vi "Seg_2_discharging.vi"(0 "VISA Refnum in":refnum<visa-resource-name>, 1 "Log??":bool, 2 "File_name":string, 5 "Numeric":i32, 7 "Index":i32, 9 "Discharge Stop Voltage":dbl=3.5 format="%#_13g", 11 "error in (no error)":errorcluster) -> (3 "Stop discharging":bool, 4 "VISA Refnum out":refnum<visa-resource-name>, 6 "Curent Tracking 2":dbl caption="Curent Tracking" format="%.8f", 10 "Voltage Tracking 2":dbl caption="Voltage Tracking" format="%.8f", 15 "error out":errorcluster)   [LabVIEW 2015]
uses:
  <vilib>/Utility/file.llb/Write Delimited Spreadsheet (string).vi
  <instrlib>/Agilent N6700 Series/Agilent N6700 Series.lvlib
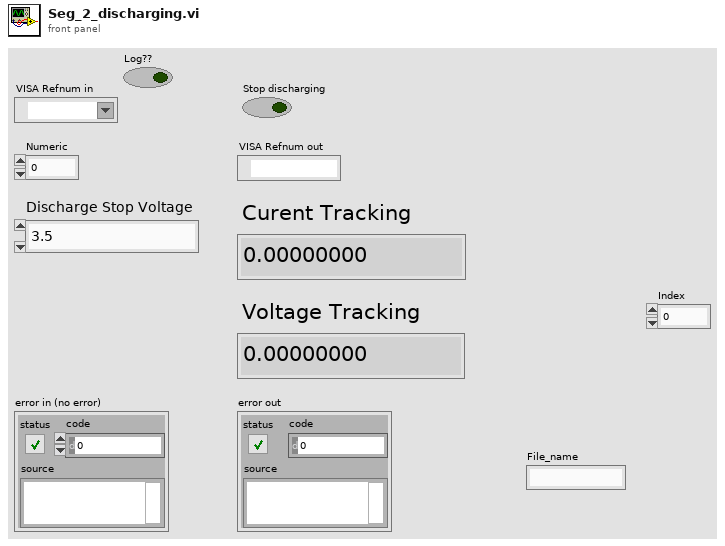
[diagram p1: front panel]
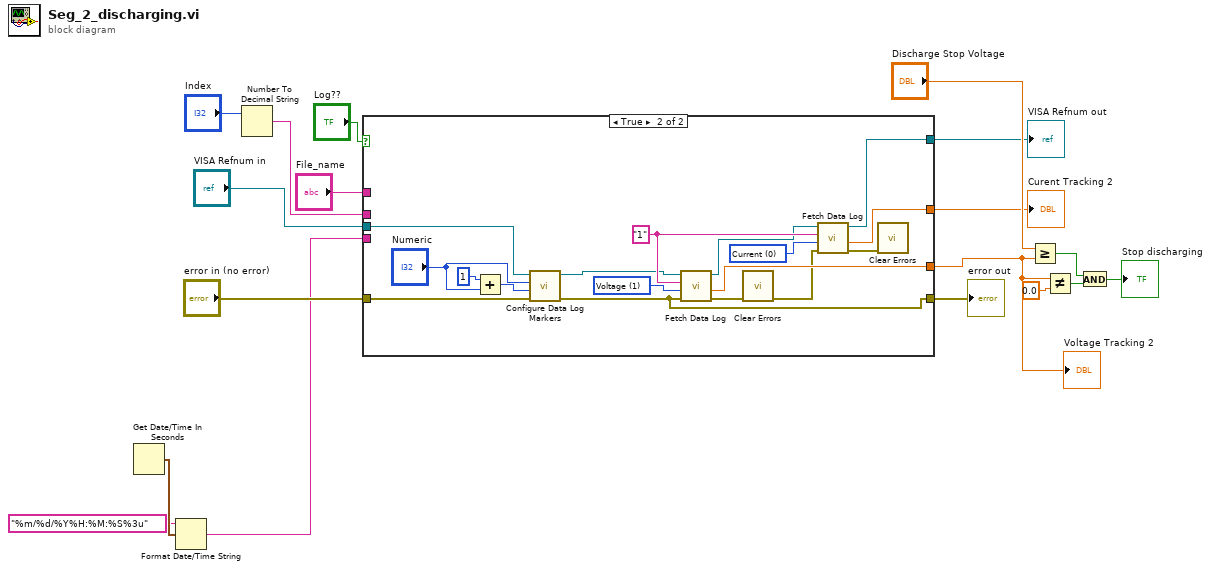
[diagram p0: block diagram]
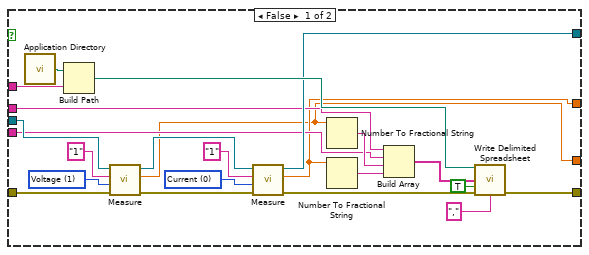
[diagram p2: hidden frame]
diagram:
  n1 = Get Date/Time In Seconds() -> (seconds since 1Jan1904=w3:timestamp)
  n2 = Format Date/Time String(time format string (%c)="%m/%d/%Y%H:%M:%S%3u", seconds (now)=w3) -> (date/time string=w1:string)  [unwired: 1 in]
  n3 = Number To Decimal String(number="Index") -> (decimal integer string=w5:string)  [unwired: 1 in]
  n4 = case shown="True" "Log??" {
    tunnel: [w20 w58] -> w18
    tunnel: [w21 w55] -> w12
    tunnel: [w27 w54] -> w11
    tunnel: [w25 w42] -> w10
    tunnel: "error in (no error)" -> [w26 w49]
    tunnel: "VISA Refnum in" -> [w28 w48]
    tunnel: w1 -> [w24 _]
    tunnel: w5 -> [w23 _]
    tunnel: "File_name" -> [w22 _]
    frame False {
      w37 = 0 items=["Current", "Voltage", "Power"] ("Measurement Type (1: Voltage)")
      w36 = 1 items=["Current", "Voltage", "Power"] ("Measurement Type (1: Voltage)")
      n5 = call <vilib>:"Application Directory.vi"() -> ("Application Directory"=w34:path)
      n6 = Build Path(base path=w34, name or relative path=w22) -> (appended path=w35:path)
      n7 = call <instrlib>:"Measure.vi"("error in (no error)"=w26, "Measurement Type (1: Voltage)"=w36, "Channel Name (1)"="1", "VISA resource name"=w28) -> ("error out"=w41:errorcluster, "Measurement"=w20:dbl, "VISA resource name out"=w40:refnum<visa-resource-name>)  [unwired: 5 in]
      n8 = call <instrlib>:"Measure.vi"("error in (no error)"=w41, "Measurement Type (1: Voltage)"=w37, "Channel Name (1)"="1", "VISA resource name"=w40) -> ("error out"=w31:errorcluster, "Measurement"=w21:dbl, "VISA resource name out"=w27:refnum<visa-resource-name>)  [unwired: 5 in]
      n9 = Number To Fractional String(number=w20) -> (F-format string=w30:string)  [unwired: 3 in]
      n10 = Number To Fractional String(number=w21) -> (F-format string=w29:string)  [unwired: 3 in]
      n11 = Build Array(w23, w24, w30, w29) -> (w32:string[])
      n12 = call-poly <vilib>:"Write Delimited Spreadsheet.vi"("file path (dialog if empty)"=w35, "1D data"=w32, "append to file? (F)"=TRUE, "error in (no error)"=w31, "delimiter (\\t)"="," ("delimiter (\\t)")) -> ("error out"=w25:errorcluster)  [unwired: 9 in, 1 out]
    }
    frame True {
      w53 = 0 items=["Voltage"=1, "Current"=0] ("Data Log Type (1: Voltage)")
      w46 = 1 items=["Voltage"=1, "Current"=0] ("Data Log Type (1: Voltage)")
      w52 = "1" ("Channel Name (1)")
      n13 = Add(x=1, y="Numeric") -> (x+y=w44:i32)
      n14 = call <instrlib>:"Configure Data Log Markers.vi"("error in (no error)"=w49, "Data Log Marker 2 (27.5 s)"=w44, "Data Log Marker 1 (7.5 s)"="Numeric", "VISA resource name"=w48) -> ("error out"=w42:errorcluster, "VISA resource name out"=w47:refnum<visa-resource-name>)  [unwired: 6 in]
      n15 = call <instrlib>:"Fetch Data Log.vi"("error in (no error)"=w42, "Data Log Type (1: Voltage)"=w46, "Channel Name (1)"=w52, "VISA resource name"=w47) -> ("error out"=w56:errorcluster, "Peak to Peak"=w58:dbl, "VISA resource name out"=w51:refnum<visa-resource-name>)  [unwired: 5 in]
      n16 = call <vilib>:"Clear Errors.vi"("error in (no error)"=w56) -> ("error out"=w43:errorcluster)  [unwired: 5 in, 1 out]
      n17 = call <instrlib>:"Fetch Data Log.vi"("error in (no error)"=w43, "Data Log Type (1: Voltage)"=w53, "Channel Name (1)"=w52, "VISA resource name"=w51) -> ("error out"=w57:errorcluster, "Peak to Peak"=w55:dbl, "VISA resource name out"=w54:refnum<visa-resource-name>)  [unwired: 5 in]
      n18 = call <vilib>:"Clear Errors.vi"("error in (no error)"=w57) -> ()  [unwired: 5 in, 2 out]
    }
  }
  "Voltage Tracking 2" <- w18
  "Curent Tracking 2" <- w12
  "VISA Refnum out" <- w11
  "error out" <- w10
  n19 = Greater Or Equal?(x="Discharge Stop Voltage", y=w18) -> (x >= y?=w14:bool)
  n20 = Not Equal?(x=w18, y=0.0) -> (x != y?=w15:bool)
  n21 = And(x=w14, y=w15) -> (x .and. y?=→"Stop discharging":bool)
